vi "Simulator SNA Resample N Complex Waveforms (Single Shot Linear Interpolation).vi"(7 "open interval? (T)":bool=TRUE, 8 "error in (no error)":errorcluster, 9 "t0":timestamp=timestamp(-9223372036854775808 s since 1904-01-01) format="%<%.4X>T", 10 "dt":dbl=1.0 format="%.2p", 11 "waveforms in":waveform(cdb)[](array[waveform])) -> (0 "error out":errorcluster, 1 "used t0's":timestamp[](array[timestamp]) format="%<%.4X>T", 3 "resampled waveforms out":waveform(cdb)[](array[waveform]), 4 "t0 adjusted warnings":bool[](array[boolean]))   [LabVIEW 2011]
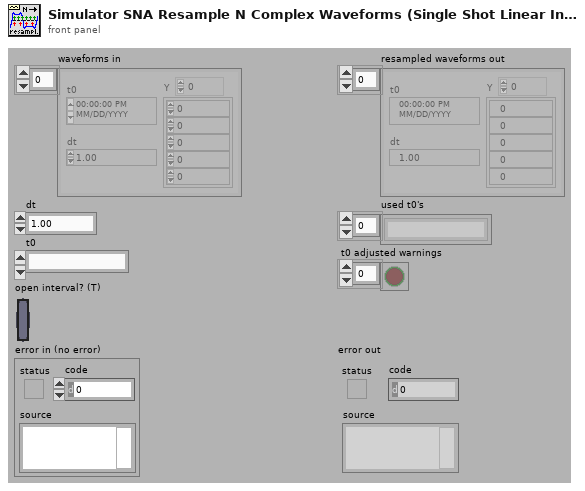
[diagram p1: front panel]
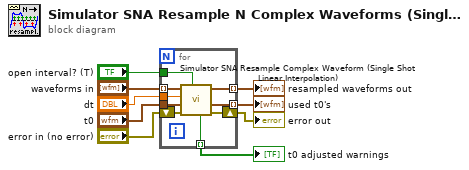
[diagram p0: block diagram]
diagram:
  n1 = for {
    tunnel: "waveforms in" -> [w18] mode=indexing
    shift-right: [w16] -> w8
    shift-left: "error in (no error)" -> [w17]
    tunnel: [w15] -> w7 mode=indexing
    tunnel: [w14] -> w6 mode=indexing
    tunnel: [w13] -> w5 mode=indexing
    tunnel: "dt" -> [w12]
    tunnel: "t0" -> [w11]
    tunnel: "open interval? (T)" -> [w10]
    n2 = call "Simulator SNA Resample Complex Waveform (Single Shot Linear Interpolation).vi"("open interval? (T)"=w10, "error in (no error)"=w17, "t0"=w11, "dt"=w12, "waveform in"=w18) -> ("error out"=w16:errorcluster, "used t0"=w15:timestamp, "resampled waveform out"=w14:waveform(cdb), "t0 adjusted warning"=w13:bool)  [unwired: 3 out]
  }
  "error out" <- w8
  "resampled waveforms out" <- w6
  "used t0's" <- w7
  "t0 adjusted warnings" <- w5
